vi "0xE1_Cmd_write_one_parameter_of_type_float_(SubVI).vi"(9 "Значение параметра":sgl, 10 "Номер параметра":i32, 11 "String in":string) -> (3 "String out":string)   [LabVIEW 2017, in "LV_Unicorn.lvlib"]
uses:
  LV_Unicorn.lvlib
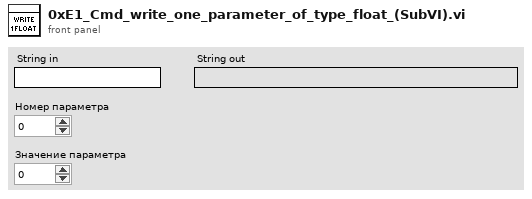
[diagram p1: front panel]
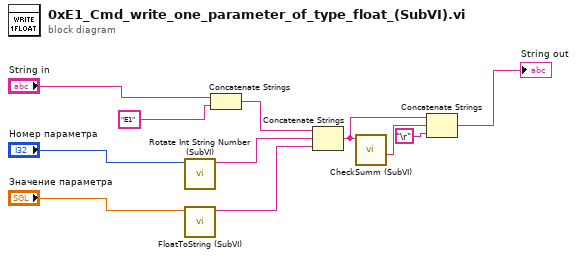
[diagram p0: block diagram]
diagram:
  n1 = call "Rotate Int String Number (SubVI).vi"("Int Number In"="Номер параметра") -> ("Orig String"=w4:string)  [unwired: 8 in, 2 out]
  n2 = call "FloatToString (SubVI).vi"("Numeric"="Значение параметра") -> ("String"=w2:string)  [unwired: 10 in]
  n3 = Concatenate Strings("String in", "E1" ("string")) -> (w9:string)
  n4 = Concatenate Strings(w9, w4, w2) -> (w6:string)
  n5 = call "CheckSumm (SubVI).vi"("Input String"=w6) -> ("CheckSumm"=w5:string)  [unwired: 7 in, 3 out]
  n6 = Concatenate Strings(w6, w5, "\r") -> (→"String out":string)
